vi "Write Multi U64.vi"(8 "error in (no error)":errorcluster, 9 "U64's":u64[](array[numeric]), 10 "Tag":string[](array[string]), 11 "Omni_Bus in":refnum<class "Omni_Bus.lvclass">) -> (0 "error out":errorcluster, 3 "Omni_Bus out":refnum<class "Omni_Bus.lvclass">)   [LabVIEW 2021, in "Omni_Bus.lvclass"]
uses:
  Omni_Bus.lvclass
  Omni_Bus.lvclass/Omni_Bus.ctl
  <vilib>/TSA/Abstract Data Classes/Abs_Types/U64 Integer/Abs_U64 Integer.lvclass
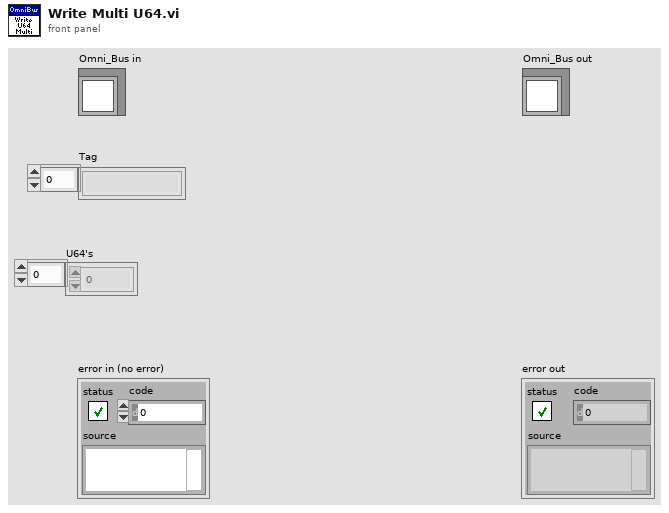
[diagram p1: front panel]
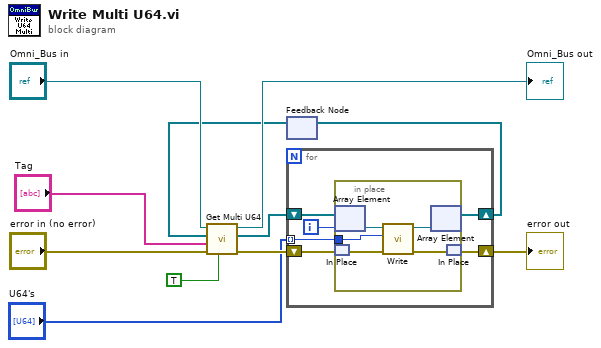
[diagram p0: block diagram]
diagram:
  n1 = feedback #1() -> (w7:refnum<class "Abs_U64 Integer.lvclass">[])  [unwired: 1 in]
  n2 = call-dynamic "Get Multi U64.vi"("Write?"=TRUE, "error in (no error)"="error in (no error)", "Tag"="Tag", "Value Type"=w7, "Var Bus in"="Omni_Bus in") -> ("error out"=w5:errorcluster, "Value Out"=w4:refnum<class "Abs_U64 Integer.lvclass">[], "Var Bus out"=→"Omni_Bus out":refnum<class "Omni_Bus.lvclass">)  [unwired: 4 in]
  n3 = for {
    tunnel: "U64's" -> [w17] mode=indexing
    shift-right: [w12] -> w1
    shift-left: w5 -> [w13]
    shift-right: [w15] -> w2
    shift-left: w4 -> [w16]
    i -> [w14]
    n4 = in-place {
      in-place-border: w17 -> [w22]
      n5 = in-place-array #2(w16, w14) -> (w21:refnum<class "Abs_U64 Integer.lvclass">)
      n6 = in-place-match #3(w13) -> (w19:errorcluster)
      n7 = call-dynamic "Write.vi"("error in (no error)"=w19, "Value"=w22, "Double Float.lvclass_340760 in"=w21) -> ("error out"=w18:errorcluster, "Double Float.lvclass_340760 out"=w20:refnum<class "Abs_U64 Integer.lvclass">)  [unwired: 7 in]
      n8 = in-place-array #2(w20) -> (w15:refnum<class "Abs_U64 Integer.lvclass">[])  [unwired: 1 out]
      n9 = in-place-match #3(w18) -> (w12:errorcluster)
    }
  }
  "error out" <- w1
  n10 = feedback-in #1(w2) -> ()
